vi "492x337.vi"() -> ()   [LabVIEW 2025]
panel:
  in  "VISA resource name out":refnum<visa-resource-name>
  in  "VISA resource name":refnum<visa-resource-name>
  out "error out":errorcluster
  in  "error in (no error)":errorcluster
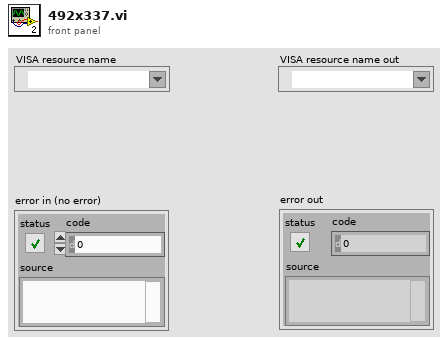
[diagram p1: front panel]
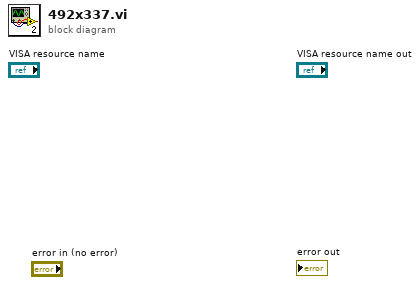
[diagram p0: block diagram]
diagram:
